vi "Write configuration.vi"(8 "error in":errorcluster, 10 "configuration":refnum<class "NISE_CEF_serializable configuration.lvclass">, 11 "RIO Target in":refnum<class "RIO Target.lvclass">) -> (0 "error out":errorcluster, 3 "RIO Target out":refnum<class "RIO Target.lvclass">)   [LabVIEW 2014, in "RIO Target.lvclass"]
uses:
  RIO Target.lvclass
  <vilib>/NI/Configuration Framework/serializable configuration/NISE_CEF_serializable configuration.lvclass
  RIO Target Configuration/RIO Target Configuration.lvclass
  RIO Target.lvclass/RIO Target.ctl
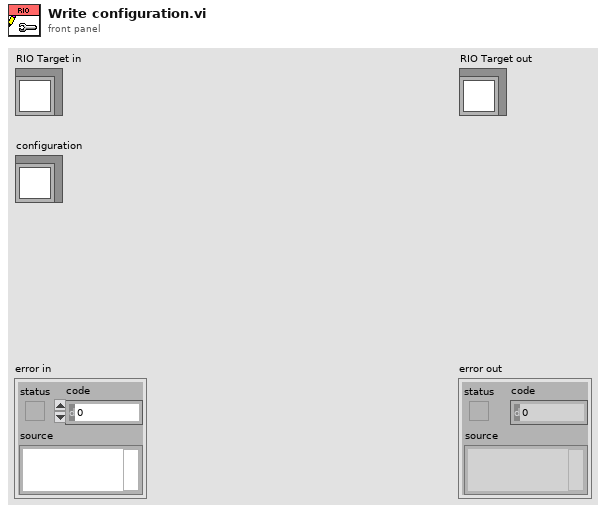
[diagram p1: front panel]
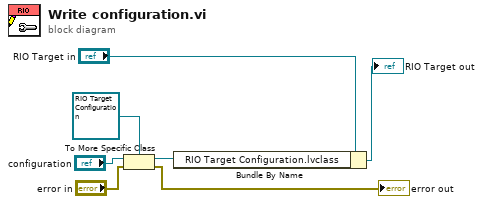
[diagram p0: block diagram]
diagram:
  n1 = To More Specific Class(target class=refnum<class "RIO Target Configuration.lvclass"> refnum ("RIO Target Configuration.lvclass"), reference="configuration", error in="error in") -> (specific class reference=w2:refnum<class "RIO Target Configuration.lvclass">, error out=→"error out":errorcluster)
  n2 = Bundle By Name(cluster="RIO Target in", "RIO Target Configuration.lvclass"=w2) -> (→"RIO Target out":refnum<class "RIO Target.lvclass">)
